vi "Shooting PID v2.vi"(11 "Setpoint":dbl) -> (0 "Output":dbl)   [LabVIEW 2016]
uses:
  Robot Global Data.vi
  <vilib>/addons/control/pid/pid.llb/PID (DBL).vi
  <vilib>/Rock Robotics/Network Tables/NT Read Numeric Array.vi
  <vilib>/addons/control/pid/NI_PID_pid.lvlib
panel:
  in  "Enable Manual":bool
  in  "Manual Setpoint":dbl=4000.0
  in  "Ramp up Interval":dbl=0.002 format="%#_13g"
  out "Rampup Complete?":bool
  in  "PID gains":T1={"proportional gain (Kc)"=0.019, "integral time (Ti, min)"=0.0, "derivative time (Td, min)"=0.0} {"derivative time (Td, min)" format="%.3f"; "integral time (Ti, min)" format="%.3f"; "proportional gain (Kc)" format="%.3f"}
  # "Does nothing, only used as a template for the incoming values from DB"
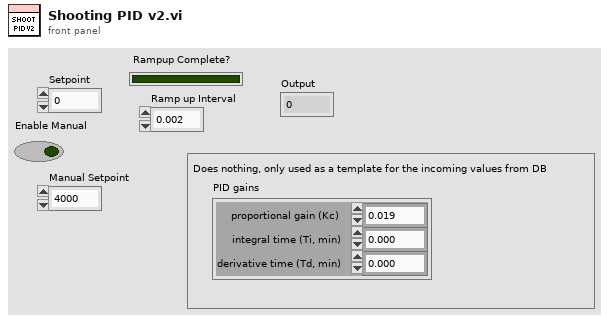
[diagram p1: front panel]
types:
  T1 = cluster{"proportional gain (Kc)":dbl, "integral time (Ti, min)":dbl, "derivative time (Td, min)":dbl}
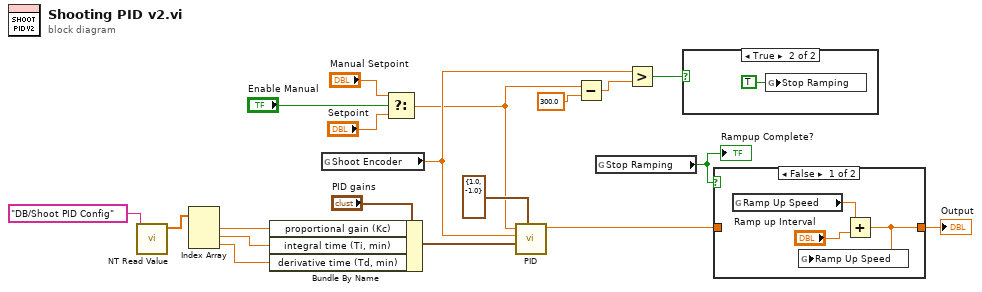
[diagram p0: block diagram]
diagram:
  n1 = call-poly <vilib>:"NT Read Value.vi"("Name"="DB/Shoot PID Config") -> ("Numeric Array"=w16:dbl[])  [unwired: 9 in, 1 out]
  n2 = Index Array(array=w16) -> (element #1=w17:dbl, element #2=w15:dbl, element #3=w14:dbl)  [unwired: 3 in]
  n3 = Bundle By Name(cluster="PID gains", "proportional gain (Kc)"=w17, "integral time (Ti, min)"=w15, "derivative time (Td, min)"=w14) -> (w13:T1)
  n4 = global read "Robot Global Data.vi" "Shoot Encoder"() -> (w9:dbl)
  n5 = Select(t="Manual Setpoint", s="Enable Manual", f="Setpoint") -> (s? t:f=w3:dbl)
  n6 = call-poly <vilib>:"PID.vi"("output range"=cluster{"output high":dbl, "output low":dbl} {"output high"=1.0, "output low"=-1.0}, "PID gains"=w13, "process variable"=w9, "setpoint"=w3) -> ("output"=w10:dbl)  [unwired: 6 in, 1 out]
  n7 = Subtract(x=w3, y=300.0) -> (x-y=w8:dbl)
  n8 = global read "Robot Global Data.vi" "Stop Ramping"() -> (w4:bool)
  "Rampup Complete?" <- w4
  n9 = Greater?(x=w9, y=w8) -> (0:w5:bool)
  n10 = case shown="True" w5 {
    frame False {
    }
    frame True {
      n11 = global write "Robot Global Data.vi" "Stop Ramping"(TRUE ("Stop Ramping")) -> ()
    }
  }
  n12 = case shown="False" w4 {
    tunnel: [w22 w24] -> w11
    tunnel: w10 -> [_ w24]
    frame False {
      n13 = global read "Robot Global Data.vi" "Ramp Up Speed"() -> (w23:dbl)
      n14 = Add(x=w23, y="Ramp up Interval") -> (x+y=w22:dbl)
      n15 = global write "Robot Global Data.vi" "Ramp Up Speed"(w22) -> ()
    }
    frame True {
    }
  }
  "Output" <- w11
